vi "Is Path a String or Array of Strings.vi"(8 "error in":errorcluster, 10 "Paths?":variant) -> (0 "error out":errorcluster, 2 "Paths.":string[](array[string]))   [LabVIEW 2020, in "Data.PG.lvclass"]
uses:
  Data.PG.lvclass
  <vilib>/Utility/error.llb/Error Cluster From Error Code.vi
  <vilib>/ErrorRing/Error Ring.xnode
  <vilib>/Utility/Data Type/NI_Data Type.lvlib
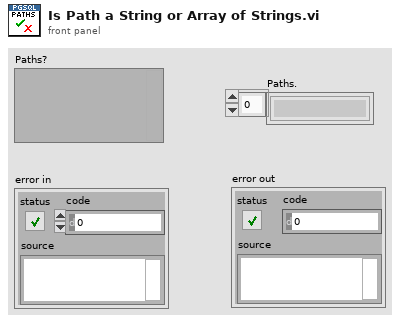
[diagram p1: front panel]
types:
  T1 = typedef "NI_Data Type.lvlib/Data Type.ctl" = enum8{"Invalid Type", "Void", "I8", "I16", "I32", "I64", "U8", "U16", "U32", "U64", "Single Float", "Double Float", "Extended Float", "Single Complex", "Double Complex", "Extended Complex", "Enum U8", "Enum U16", "Enum U32", "Enum U64", "Single Float With Unit", "Double Float With Unit", "Extended Float With Unit", "Single Complex with Unit", "Double Complex with Unit", "Extended Complex with Unit", "Boolean", "String", "Path", "Picture", "Tag", "Array", "Cluster", "Variant", "LV Variant", "Waveform", "Timestamp", "Digital Waveform", "Digital Data", "ExpressData", "Refnum", "External Data", "VI", "Poly VI", "LabVIEW Class Instance", "Fixed Point", "Set Collection", "Map Collection"}
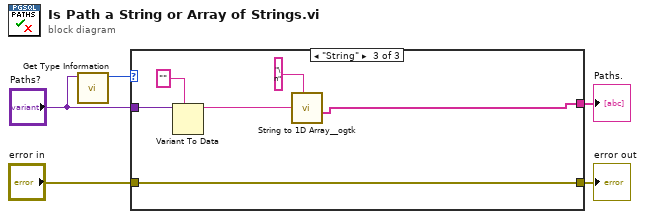
[diagram p0: block diagram]
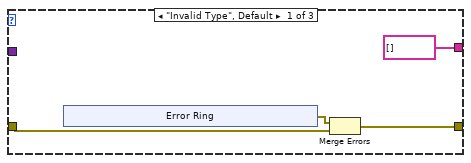
[diagram p2: hidden frame]
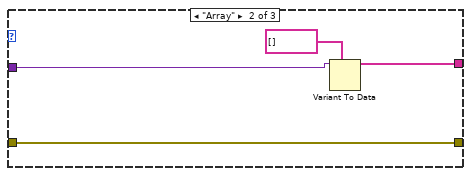
[diagram p3: hidden frame]
diagram:
  n1 = call <vilib>:"Get Type Information.vi"("variant"="Paths?") -> ("type"=w5:T1)  [unwired: 6 in, 4 out]
  n2 = case shown="\"String\"" w5 {
    tunnel: "Paths?" -> [_ w18 w23]
    tunnel: [string[] [] w16 w20] -> w2
    tunnel: "error in" -> [w8 w15 w22]
    tunnel: [w6 w15 w22] -> w1
    frame "Invalid Type", Default {
      n3 = xnode "Error Ring"() -> ("error out"=w7:errorcluster)
      n4 = Merge Errors(w7, w8) -> (w6:errorcluster)
    }
    frame "Array" {
      n5 = Variant To Data(type=string[] [], Variant=w18) -> (data=w16:string[])  [unwired: 1 in, 1 out]
    }
    frame "String" {
      n6 = Variant To Data(type="", Variant=w23) -> (data=w21:string)  [unwired: 1 in, 1 out]
      n7 = call <userlib>:"String to 1D Array__ogtk.vi"("delimiter (Tab)"="\n", "string"=w21) -> ("Array of Strings"=w20:string[])  [unwired: 9 in]
    }
  }
  "Paths." <- w2
  "error out" <- w1
